vi "tcs shm wait For Completion Set Value LV.vi"(8 "error in (no error)":errorcluster, 11 "waitComplete_Ctl":cluster{"cmdSeqNum":i32, "timeout":u32}) -> (0 "error out":errorcluster, 2 "function return":i32, 3 "waitComplete_Ctl out":cluster{"cmdSeqNum":i32, "timeout":u32})   [LabVIEW 2016, in "SALLV_tcs.lvlib"]
doc: "int tcs_shm_waitForCompletion_SetValueLV(tcs_waitCompleteLV *waitComplete_Ctl);"
uses:
  SALLV_tcs.lvlib
  SALLV_tcs.so
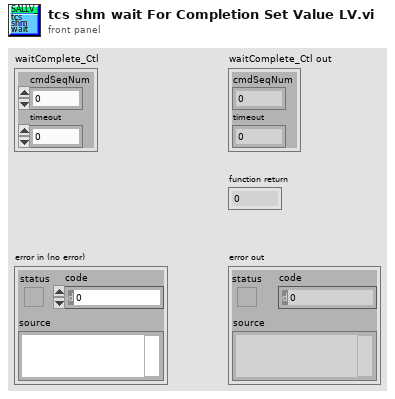
[diagram p1: front panel]
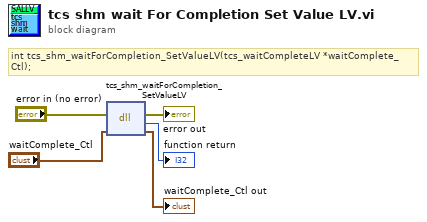
[diagram p0: block diagram]
diagram:
  # "int tcs_shm_waitForCompletion_SetValueLV(tcs_waitCompleteLV *waitComplete_Ctl);"
  n1 = dll-call lib="home/plotz/SALLV_tcs/SALLV_tcs.*" fn="tcs_shm_waitForCompletion_SetValueLV"(error in="error in (no error)", "waitComplete_Ctl"="waitComplete_Ctl") -> (error out=→"error out":errorcluster, →"function return":i32, "waitComplete_Ctl"=→"waitComplete_Ctl out":cluster{"cmdSeqNum":i32, "timeout":u32})  [unwired: 2 in, 1 out]
